vi "BMU诊断标定.vi"(5 "timeout":u32, 6 "Socket":dbl, 7 "通用配置?":bool, 8 "CAN端口":u16(ring), 9 "设备索引号":u16(ring), 10 "CAN卡类型":u32(ring)=21, 11 "从板号":u8=1) -> (3 "成功?":bool)   [LabVIEW 2013] (continued)
              n4251 = call "CAN_Init-8.6.vi"("CAN卡类型"=w6125, "设备索引号"=w6124, "CAN端口"=w6123, "操作类型"=enum16{"初始化CAN", "关闭CAN"}."初始化CAN", "滤波方式"=w6120, "Accept Code"=u32 3221225472, "簇"=T23 {"打开CAN"=FALSE, "初始化CAN"=TRUE, "开始CAN"=TRUE, "重启"=FALSE, "关闭CAN"=FALSE}, "Mask Code"=u32 1073741823 ("Accept Code"), "工作方式"=w6119, "是否滤波"=TRUE, "滤波选择"=T22 {"fiter_mode"=1, "fiter_endid"=402653184, "fiter_startid"=419430399}) -> ()  [unwired: 3 in, 6 out]
              n4252 = call <vilib>:"Unset Busy.vi"() -> ()  [unwired: 2 in, 10 out]
            }
          }
        }
        frame "强制均衡" {
          n4253 = local read "从板板号"() -> (w6129:u8)
          n4254 = stacked-sequence {
            tunnel: 133 -> [_ w6160 _ _]
            tunnel: w6129 -> [_ _ _ _]
            frame #0 {
              w6139 = u8 0 items=["Normal", "Listen Only"] ("工作方式")
              w6138 = u8 1 items=["Dual Filter", "Single Filter"] ("滤波方式")
              n4255 = global write "EV05全局变量1.vi" "读取超时"(FALSE ("读取超时")) -> ()
              n4256 = global write "EV05全局变量1.vi" "流控帧 2"(TRUE ("流控帧 2")) -> ()
              n4257 = local write "写?"(TRUE ("写?")) -> ()
              n4258 = local read "设备索引号"() -> (w6134:u16)
              n4259 = local read "CAN卡类型"() -> (w6133:u32)
              n4260 = local write "控制1"(TRUE ("控制1")) -> ()
              n4261 = local read "CAN端口"() -> (w6135:u16)
              n4262 = local write "消除"(TRUE ("消除")) -> ()
              n4263 = global write "EV05全局变量1.vi" "流控帧"(FALSE ("流控帧")) -> ()
              n4264 = call "CAN_Init-8.6.vi"("CAN卡类型"=w6133, "设备索引号"=w6134, "CAN端口"=w6135, "操作类型"=enum16{"初始化CAN", "关闭CAN"}."初始化CAN", "滤波方式"=w6138, "Accept Code"=u32 606601216, "簇"=T23 {"打开CAN"=FALSE, "初始化CAN"=TRUE, "开始CAN"=TRUE, "重启"=FALSE, "关闭CAN"=FALSE}, "Mask Code"=u32 524287 ("Accept Code"), "工作方式"=w6139, "是否滤波"=TRUE, "滤波选择"=T22 {"fiter_mode"=1, "fiter_endid"=75825152, "fiter_startid"=75890687}) -> ()  [unwired: 3 in, 6 out]
              n4265 = Wait Until Next ms Multiple(millisecond multiple=u32 20 ("毫秒倍数")) -> ()  [unwired: 1 out]
            }
            frame #1 {
              n4266 = local read "强制类型"() -> (w6166:enum16{"全通道开启", "单通道开启", "清待均衡时间"})
              n4267 = case shown="\"清待均衡时间\"" w6166 {
                tunnel: [250 252 254] -> w6156
                tunnel: [_ w6185 _] -> w6155
                tunnel: [_ w6184 _] -> w6154
                tunnel: [_ w6175 _] -> w6153
                tunnel: [_ w6168 _] -> w6152
                frame "全通道开启", Default {
                }
                frame "单通道开启" {
                  n4268 = local read "均衡类型选择"() -> (w6183:enum16{"放电均衡", "充电均衡", "充放电均衡"})
                  n4269 = local read "均衡位置"() -> (w6178:u16)
                  n4270 = case shown="\"放电均衡\", 默认" w6183 {
                    tunnel: [0 1] -> w6182
                    frame "放电均衡", Default {
                    }
                    frame "充电均衡" {
                    }
                  }
                  n4271 = Multiply(x="均衡时间", y=6.0) -> (x*y=w6170:dbl)
                  n4272 = Quotient & Remainder(x=w6170, y=256.0) -> (x-y*floor(x/y)=w6168:dbl, floor(x/y)=w6169:dbl)
                  n4273 = call "二进制解析-8.6.vi"("索引"=1, "数值"=w6182) -> ("低位子数组"=w6173:i32[])  [unwired: 1 in, 2 out]
                  n4274 = Quotient & Remainder(x=w6178, y=256.0) -> (x-y*floor(x/y)=w6184:dbl, floor(x/y)=w6185:dbl)
                  n4275 = call "二进制解析-8.6.vi"("索引"=8, "数值"=w6169) -> ("低位子数组"=w6174:i32[])  [unwired: 1 in, 2 out]
                  n4276 = Replace Array Subset(array=w6174, new element=w6173, index=0 ("索引")) -> (w6171:i32[])
                  n4277 = call "数值二进制转十进制-8.6.vi"("子数组"=w6171) -> ("十进制数值"=w6175:i32)  [unwired: 4 in]
                }
                frame "清待均衡时间" {
                }
              }
              n4278 = local write "命令"(w6160) -> ()
              n4279 = call "ID组合.vi"("SA(4)"=0 ("PDU(1)"), "PS(3)"=63 ("PDU(1)"), "PF(2)"=w6160, "PDU(1)"=4) -> ("ID"=w6159:i32)  [unwired: 7 out]
              n4280 = local read "设备索引号"() -> (w6163:u16)
              n4281 = local read "CAN卡类型"() -> (w6164:u32)
              n4282 = local read "CAN端口"() -> (w6162:u16)
              n4283 = local write "命令序号"(w6156) -> ()
              n4284 = Build Array(6, 4, w6156, w6155, w6154, w6153, w6152) -> (w6165:dbl[])
              n4285 = call "transmit-8.6.vi"("can卡类型"=w6164, "设备索引号"=w6163, "CAN端口"=w6162, "ID"=w6159, "SendType"=u8 0, "Data"=w6165) -> ()  [unwired: 3 in, 11 out]
            }
            frame #2 {
              n4286 = Wait Until Next ms Multiple(millisecond multiple=u32 1000 ("毫秒倍数")) -> ()  [unwired: 1 out]
            }
            frame #3 {
              w6199 = u8 0 items=["Normal", "Listen Only"] ("工作方式")
              w6198 = u8 1 items=["Dual Filter", "Single Filter"] ("滤波方式")
              n4287 = global write "EV05全局变量1.vi" "流控帧 2"(FALSE ("流控帧 2")) -> ()
              n4288 = local write "控制1"(FALSE ("控制1")) -> ()
              n4289 = local read "设备索引号"() -> (w6194:u16)
              n4290 = local read "CAN卡类型"() -> (w6193:u32)
              n4291 = local write "消除"(FALSE ("消除")) -> ()
              n4292 = local read "CAN端口"() -> (w6195:u16)
              n4293 = call <vilib>:"Unset Busy.vi"() -> ()  [unwired: 2 in, 10 out]
              n4294 = call "CAN_Init-8.6.vi"("CAN卡类型"=w6193, "设备索引号"=w6194, "CAN端口"=w6195, "操作类型"=enum16{"初始化CAN", "关闭CAN"}."初始化CAN", "滤波方式"=w6198, "Accept Code"=u32 3221225472, "簇"=T23 {"打开CAN"=FALSE, "初始化CAN"=TRUE, "开始CAN"=TRUE, "重启"=FALSE, "关闭CAN"=FALSE}, "Mask Code"=u32 1073741823 ("Accept Code"), "工作方式"=w6199, "是否滤波"=TRUE, "滤波选择"=T22 {"fiter_mode"=1, "fiter_endid"=402653184, "fiter_startid"=419430399}) -> ()  [unwired: 3 in, 6 out]
            }
          }
        }
        frame "项目软件版本读取" {
          n4295 = stacked-sequence {
            seq-local: [_ w6220 _] -> [_ _ w6227]
            frame #0 {
              n4296 = local read "设备索引号"() -> (w6207:u16)
              n4297 = local read "CAN卡类型"() -> (w6208:u32)
              n4298 = local read "CAN端口"() -> (w6206:u16)
              n4299 = stacked-sequence {
                tunnel: w6208 -> [w6211 w6219]
                tunnel: w6207 -> [w6210 w6218]
                tunnel: w6206 -> [w6209 w6217]
                frame #0 {
                  n4300 = dll-call lib="PTH1abs FBluewave New EnergySVN_WorkAutoTest_TestStandtrunkAutoTest_TestStandDriverZlgCanBHN01è¯»ååæ°data\nkerneldlls\nusbcan.dll" fn="VCI_ClearBuffer"("DeviceType"=w6211, "DeviceInd"=w6210, "CANInd"=w6209) -> (error out=w6212:errorcluster)  [unwired: 4 in, 4 out]
                  n4301 = call <vilib>:"Clear Errors.vi"("error in (no error)"=w6212) -> ()  [unwired: 6 in, 1 out]
                }
                frame #1 {
                  w6216 = u8 137 ("命令")
                  w6215 = u32 1 ("命令序号")
                  n4302 = local read "从板板号"() -> (w6213:u8)
                  n4303 = local write "命令"(w6216) -> ()
                  n4304 = call "多帧发送机制(EV05).vi"("can卡类型"=w6219, "设备索引号"=w6218, "CAN端口"=w6217, "命令"=w6216, "板号"=w6213, "命令序号"=w6215, "输入数据"=dbl[] [0.0]) -> ()  [unwired: 2 in, 11 out]
                  n4305 = local write "命令序号"(w6215) -> ()
                }
              }
            }
            frame #1 {
              n4306 = while {
                tunnel: [w6221] -> w6220
                i -> [w6226]
                stop <- w6223 stop-if-true
                n4307 = global read "EV05全局变量1.vi" "写入超时"() -> (w6221:bool)
                n4308 = Greater Or Equal?(x=w6226, y=25) -> (x >= y?=w6224:bool)
                n4309 = Or(x=w6221, y=w6224) -> (x .or. y?=w6223:bool)
                n4310 = Wait Until Next ms Multiple(millisecond multiple=u32 100 ("毫秒倍数")) -> ()  [unwired: 1 out]
              }
            }
            frame #2 {
              n4311 = case shown="假" w6227 {
                frame False {
                  n4312 = control-ref of="结果"() -> (w6229:refnum<vi>)
                  n4313 = Concatenate Strings("项目软件版本" ("字符串"), "     读取失败" ("字符串")) -> (w6232:string)
                  n4314 = Build Array(w6232) -> (w6231:string[])
                  n4315 = call "表格编辑(版本读取).vi"("新元素/子数组"=w6231, "活动单元格:单元格背景色"=u32 16740749, "MCListbox引用句柄"=w6229) -> ()  [unwired: 9 out]
                }
                frame True {
                }
              }
              n4316 = call <vilib>:"Unset Busy.vi"() -> ()  [unwired: 2 in, 10 out]
            }
          }
        }
        frame "读取故障状态" {
          n4317 = stacked-sequence {
            seq-local: [_ w6258 _] -> [_ _ w6265]
            frame #0 {
              n4318 = local read "设备索引号"() -> (w6235:u16)
              n4319 = local read "CAN卡类型"() -> (w6236:u32)
              n4320 = local read "CAN端口"() -> (w6234:u16)
              n4321 = stacked-sequence {
                tunnel: w6236 -> [w6239 w6248]
                tunnel: w6235 -> [w6238 w6247]
                tunnel: w6234 -> [w6237 w6246]
                frame #0 {
                  n4322 = dll-call lib="PTH1abs FBluewave New EnergySVN_WorkAutoTest_TestStandtrunkAutoTest_TestStandDriverZlgCanBHN01è¯»ååæ°data\nkerneldlls\nusbcan.dll" fn="VCI_ClearBuffer"("DeviceType"=w6239, "DeviceInd"=w6238, "CANInd"=w6237) -> (error out=w6240:errorcluster)  [unwired: 4 in, 4 out]
                  n4323 = call <vilib>:"Clear Errors.vi"("error in (no error)"=w6240) -> ()  [unwired: 6 in, 1 out]
                }
                frame #1 {
                  n4324 = local read "从板板号 2"() -> (w6241:u8)
                  n4325 = case shown="1..30" w6241 {
                    tunnel: [u8 133 ("命令") u8 4 ("命令")] -> w6245
                    frame 0, Default {
                    }
                    frame 1..30 {
                    }
                  }
                  n4326 = local read "状态选择"() -> (w6243:T18)
                  n4327 = local write "命令"(w6245) -> ()
                  n4328 = case shown="\"预充电故障,继电器驱动故障\"" w6243 {
                    tunnel: [1 2 3 4 5 6 7] -> w6242
                    frame "电压,内总电压,外总电压,温度,电流,绝缘,系统时钟,充电均衡,放电均衡", Default {
                    }
                    frame "CPU,CPU内部EE存储器,CPU内部FLASH,内部EE存储器,45db存储器" {
                    }
                    frame "CAN检测故障" {
                    }
                    frame "软件故障" {
                    }
                    frame "RS485,RS232检测故障" {
                    }
                    frame "DI,DO,AI,AO检测故障" {
                    }
                    frame "预充电故障,继电器驱动故障" {
                    }
                  }
                  n4329 = call "多帧发送机制(EV05).vi"("can卡类型"=w6248, "设备索引号"=w6247, "CAN端口"=w6246, "命令"=w6245, "板号"=w6241, "命令序号"=w6242, "输入数据"=dbl[] [0.0]) -> ()  [unwired: 2 in, 11 out]
                  n4330 = local write "命令序号"(w6242) -> ()
                }
              }
            }
            frame #1 {
              n4331 = while {
                tunnel: [w6259] -> w6258
                i -> [w6264]
                stop <- w6261 stop-if-true
                n4332 = global read "EV05全局变量1.vi" "写入超时"() -> (w6259:bool)
                n4333 = Greater Or Equal?(x=w6264, y=25) -> (x >= y?=w6262:bool)
                n4334 = Or(x=w6259, y=w6262) -> (x .or. y?=w6261:bool)
                n4335 = Wait Until Next ms Multiple(millisecond multiple=u32 100 ("毫秒倍数")) -> ()  [unwired: 1 out]
              }
            }
            frame #2 {
              n4336 = case shown="真" w6265 {
                frame False {
                  n4337 = Concatenate Strings("故障信息" ("字符串"), "     读取失败" ("字符串")) -> (w6267:string)
                  n4338 = One Button Dialog(message=w6267, button name ("OK")="确定" ("按钮名称（“确定”）")) -> ()  [unwired: 1 out]
                }
                frame True {
                  n4339 = One Button Dialog(message="故障信息读取完成" ("字符串"), button name ("OK")="确定" ("按钮名称（“确定”）")) -> ()  [unwired: 1 out]
                }
              }
              n4340 = call <vilib>:"Unset Busy.vi"() -> ()  [unwired: 2 in, 10 out]
            }
          }
        }
        frame "平台软件版本读取" {
          n4341 = stacked-sequence {
            seq-local: [_ w6287 _] -> [_ _ w6294]
            frame #0 {
              n4342 = local read "设备索引号"() -> (w6274:u16)
              n4343 = local read "CAN卡类型"() -> (w6275:u32)
              n4344 = local read "CAN端口"() -> (w6273:u16)
              n4345 = stacked-sequence {
                tunnel: w6275 -> [w6278 w6286]
                tunnel: w6274 -> [w6277 w6285]
                tunnel: w6273 -> [w6276 w6284]
                tunnel: u8 137 ("命令") -> [_ w6283]
                frame #0 {
                  n4346 = dll-call lib="PTH1abs FBluewave New EnergySVN_WorkAutoTest_TestStandtrunkAutoTest_TestStandDriverZlgCanBHN01è¯»ååæ°data\nkerneldlls\nusbcan.dll" fn="VCI_ClearBuffer"("DeviceType"=w6278, "DeviceInd"=w6277, "CANInd"=w6276) -> (error out=w6279:errorcluster)  [unwired: 4 in, 4 out]
                  n4347 = call <vilib>:"Clear Errors.vi"("error in (no error)"=w6279) -> ()  [unwired: 6 in, 1 out]
                }
                frame #1 {
                  w6282 = u32 2 ("命令序号")
                  n4348 = local read "从板板号"() -> (w6280:u8)
                  n4349 = local write "命令"(w6283) -> ()
                  n4350 = call "多帧发送机制(EV05).vi"("can卡类型"=w6286, "设备索引号"=w6285, "CAN端口"=w6284, "命令"=w6283, "板号"=w6280, "命令序号"=w6282, "输入数据"=dbl[] [0.0]) -> ()  [unwired: 2 in, 11 out]
                  n4351 = local write "命令序号"(w6282) -> ()
                }
              }
            }
            frame #1 {
              n4352 = while {
                tunnel: [w6288] -> w6287
                i -> [w6293]
                stop <- w6290 stop-if-true
                n4353 = global read "EV05全局变量1.vi" "写入超时"() -> (w6288:bool)
                n4354 = Greater Or Equal?(x=w6293, y=25) -> (x >= y?=w6291:bool)
                n4355 = Or(x=w6288, y=w6291) -> (x .or. y?=w6290:bool)
                n4356 = Wait Until Next ms Multiple(millisecond multiple=u32 100 ("毫秒倍数")) -> ()  [unwired: 1 out]
              }
            }
            frame #2 {
              n4357 = case shown="假" w6294 {
                frame False {
                  n4358 = control-ref of="结果"() -> (w6297:refnum<vi>)
                  n4359 = Concatenate Strings("平台软件版本" ("字符串"), "     读取失败" ("字符串")) -> (w6299:string)
                  n4360 = Build Array(w6299) -> (w6296:string[])
                  n4361 = call "表格编辑(版本读取).vi"("新元素/子数组"=w6296, "活动单元格:单元格背景色"=u32 16740749, "MCListbox引用句柄"=w6297) -> ()  [unwired: 9 out]
                }
                frame True {
                }
              }
              n4362 = call <vilib>:"Unset Busy.vi"() -> ()  [unwired: 2 in, 10 out]
            }
          }
        }
        frame "模块软件版本读取" {
          n4363 = local read "从板板号"() -> (w6301:u8)
          n4364 = local read "模块软件版本"() -> (w6302:T1)
          n4365 = case shown="\"全部读取\"" w6302 {
            selector: w6302 -> [w6303 w6347]
            tunnel: w6301 -> [_ w6346]
            frame "BCUMCAL", Default {
              n4366 = stacked-sequence {
                seq-local: [_ _ w6329 _] -> [_ _ _ w6336]
                tunnel: w6303 -> [_ w6309 _ w6337]
                frame #0 {
                  w6308 = FALSE ("写?")
                  n4367 = call <vilib>:"Set Busy.vi"("disable click? (T)"=FALSE) -> ()  [unwired: 3 in, 8 out]
                  n4368 = local write "写?"(w6308) -> ()
                  n4369 = global write "EV05全局变量1.vi" "流控帧 2"(TRUE ("流控帧 2")) -> ()
                  n4370 = global write "EV05全局变量1.vi" "写入超时"(w6308) -> ()
                  n4371 = local write "控制1"(TRUE ("控制1")) -> ()
                  n4372 = local write "消除"(TRUE ("消除")) -> ()
                }
                frame #1 {
                  n4373 = Quotient & Remainder(x=w6309, y=256) -> (x-y*floor(x/y)=w6310:i32, floor(x/y)=w6311:i32)
                  n4374 = Build Array(w6311, w6310, u8 0 ("板号")) -> (w6314:i32[])
                  n4375 = local read "设备索引号"() -> (w6316:u16)
                  n4376 = local read "CAN卡类型"() -> (w6317:u32)
                  n4377 = local read "CAN端口"() -> (w6315:u16)
                  n4378 = stacked-sequence {
                    tunnel: w6317 -> [w6320 w6328]
                    tunnel: w6316 -> [w6319 w6327]
                    tunnel: w6315 -> [w6318 w6326]
                    tunnel: w6314 -> [_ w6325]
                    frame #0 {
                      n4379 = dll-call lib="PTH1abs FBluewave New EnergySVN_WorkAutoTest_TestStandtrunkAutoTest_TestStandDriverZlgCanBHN01è¯»ååæ°data\nkerneldlls\nusbcan.dll" fn="VCI_ClearBuffer"("DeviceType"=w6320, "DeviceInd"=w6319, "CANInd"=w6318) -> (error out=w6321:errorcluster)  [unwired: 4 in, 4 out]
                      n4380 = call <vilib>:"Clear Errors.vi"("error in (no error)"=w6321) -> ()  [unwired: 6 in, 1 out]
                    }
                    frame #1 {
                      w6324 = u8 137 ("命令")
                      w6322 = u32 3 ("命令序号")
                      n4381 = local read "从板板号"() -> (w6323:u8)
                      n4382 = local write "命令"(w6324) -> ()
                      n4383 = call "多帧发送机制(EV05).vi"("can卡类型"=w6328, "设备索引号"=w6327, "CAN端口"=w6326, "命令"=w6324, "板号"=w6323, "命令序号"=w6322, "输入数据"=w6325) -> ()  [unwired: 2 in, 11 out]
                      n4384 = local write "命令序号"(w6322) -> ()
                    }
                  }
                }
                frame #2 {
                  n4385 = while {
                    tunnel: [w6330] -> w6329
                    i -> [w6335]
                    stop <- w6331 stop-if-true
                    n4386 = global read "EV05全局变量1.vi" "写入超时"() -> (w6330:bool)
                    n4387 = Greater Or Equal?(x=w6335, y=25) -> (x >= y?=w6332:bool)
                    n4388 = Or(x=w6330, y=w6332) -> (x .or. y?=w6331:bool)
                    n4389 = Wait Until Next ms Multiple(millisecond multiple=u32 100 ("毫秒倍数")) -> ()  [unwired: 1 out]
                  }
                }
                frame #3 {
                  n4390 = call <vilib>:"Unset Busy.vi"() -> ()  [unwired: 2 in, 10 out]
                  n4391 = case shown="假" w6336 {
                    tunnel: w6337 -> [w6339 _]
                    frame False {
                      n4392 = Number To Decimal String(number=w6339) -> (decimal integer string=w6340:string)  [unwired: 1 out]
                      n4393 = control-ref of="结果"() -> (w6341:refnum<vi>)
                      n4394 = Concatenate Strings("模块" ("字符串"), w6340, "     读取失败" ("字符串")) -> (w6344:string)
                      n4395 = Build Array(w6344) -> (w6343:string[])
                      n4396 = call "表格编辑(版本读取).vi"("新元素/子数组"=w6343, "活动单元格:单元格背景色"=u32 16740749, "MCListbox引用句柄"=w6341) -> ()  [unwired: 9 out]
                    }
                    frame True {
                    }
                  }
                }
              }
            }
            frame "全部读取" {
              n4397 = stacked-sequence {
                seq-local: [w6348 _] -> [_ w6386]
                tunnel: w6347 -> [_ w6388]
                tunnel: w6346 -> [w6349 w6387]
                frame #0 {
                  n4398 = stacked-sequence {
                    tunnel: w6349 -> [_ w6358 _]
                    tunnel: [_ _ w6378] -> w6348
                    frame #0 {
                      w6354 = FALSE ("写?")
                      n4399 = control-ref of="模块软件版本 2"() -> (w6352:refnum<vi>)
                      n4400 = call <vilib>:"Set Busy.vi"("disable click? (T)"=FALSE) -> ()  [unwired: 3 in, 8 out]
                      n4401 = local write "写?"(w6354) -> ()
                      n4402 = property class="MCListbox (严格)"(reference=w6352, "ItemNames"=string[][] []) -> ()  [unwired: 1 in, 2 out]
                      n4403 = global write "EV05全局变量1.vi" "写入超时"(w6354) -> ()
                      n4404 = local write "消除"(TRUE ("消除")) -> ()
                      n4405 = global write "EV05全局变量1.vi" "流控帧 2"(TRUE ("流控帧 2")) -> ()
                      n4406 = local write "控制1"(TRUE ("控制1")) -> ()
                      n4407 = local write "MODEL号"(u8[] [] ("MODEL号")) -> ()
                    }
                    frame #1 {
                      n4408 = local read "设备索引号"() -> (w6360:u16)
                      n4409 = local read "CAN卡类型"() -> (w6361:u32)
                      n4410 = local read "CAN端口"() -> (w6359:u16)
                      n4411 = stacked-sequence {
                        tunnel: w6361 -> [w6364 w6377]
                        tunnel: w6360 -> [w6363 w6376]
                        tunnel: w6359 -> [w6362 w6375]
                        tunnel: w6358 -> [_ w6367]
                        frame #0 {
                          n4412 = dll-call lib="PTH1abs FBluewave New EnergySVN_WorkAutoTest_TestStandtrunkAutoTest_TestStandDriverZlgCanBHN01è¯»ååæ°data\nkerneldlls\nusbcan.dll" fn="VCI_ClearBuffer"("DeviceType"=w6364, "DeviceInd"=w6363, "CANInd"=w6362) -> (error out=w6365:errorcluster)  [unwired: 4 in, 4 out]
                          n4413 = call <vilib>:"Clear Errors.vi"("error in (no error)"=w6365) -> ()  [unwired: 6 in, 1 out]
                        }
                        frame #1 {
                          w6373 = u8 137 ("命令")
                          w6371 = u32 3 ("命令序号")
                          n4414 = Quotient & Remainder(x=u8 0 ("板号"), y=256) -> (x-y*floor(x/y)=w6368:i32, floor(x/y)=w6369:i32)
                          n4415 = local write "命令"(w6373) -> ()
                          n4416 = Build Array(w6369, w6368, u8 0 ("板号")) -> (w6374:i32[])
                          n4417 = call "多帧发送机制(EV05).vi"("can卡类型"=w6377, "设备索引号"=w6376, "CAN端口"=w6375, "命令"=w6373, "板号"=w6367, "命令序号"=w6371, "输入数据"=w6374) -> ()  [unwired: 2 in, 11 out]
                          n4418 = local write "命令序号"(w6371) -> ()
                        }
                      }
                    }
                    frame #2 {
                      n4419 = while {
                        tunnel: [w6380] -> w6378
                        i -> [w6384]
                        stop <- w6381 stop-if-true
                        n4420 = local read "强制停止版本读取"() -> (w6379:bool)
                        n4421 = global read "EV05全局变量1.vi" "写入超时"() -> (w6380:bool)
                        n4422 = Greater Or Equal?(x=w6384, y=35) -> (x >= y?=w6382:bool)
                        n4423 = Compound Arithmetic op=OR(w6379, w6380, w6382) -> (w6381:bool)
                        n4424 = Wait Until Next ms Multiple(millisecond multiple=u32 100 ("毫秒倍数")) -> ()  [unwired: 1 out]
                      }
                    }
                  }
                }
                frame #1 {
                  n4425 = case shown="真" w6386 {
                    tunnel: w6388 -> [_ w6398]
                    tunnel: w6387 -> [_ w6397]
                    frame False {
                      n4426 = control-ref of="结果"() -> (w6390:refnum<vi>)
                      n4427 = Concatenate Strings("模块编号" ("字符串"), "读取失败" ("字符串")) -> (w6393:string)
                      n4428 = Build Array(w6393) -> (w6392:string[])
                      n4429 = call "表格编辑(版本读取).vi"("新元素/子数组"=w6392, "活动单元格:单元格背景色"=u32 16740749, "MCListbox引用句柄"=w6390) -> ()  [unwired: 9 out]
                      n4430 = call <vilib>:"Unset Busy.vi"() -> ()  [unwired: 11 in, 1 out]
                    }
                    frame True {
                      n4431 = local read "MODEL号"() -> (w6396:u8[])
                      n4432 = Array Size(array=w6396) -> (size(s)=w6395:i32)
                      n4433 = for {
                        tunnel: w6398 -> [_]
                        tunnel: w6397 -> [w6401]
                        tunnel: w6396 -> [w6400] mode=indexing
                        tunnel: w6395 -> [w6399]
                        i -> [w6403]
                        n4434 = Increment(x=w6403) -> (x+1=w6402:i32)
                        n4435 = stacked-sequence {
                          seq-local: [_ _ _ w6430 _ _] -> [_ _ _ _ w6439 _]
                          seq-local: [_ w6409 _ _ _ _] -> [_ _ _ _ w6438 _]
                          tunnel: w6402 -> [_ _ _ _ _ w6450]
                          tunnel: w6400 -> [_ w6409 _ _ _ _]
                          tunnel: w6401 -> [_ w6410 _ _ _ _]
                          tunnel: w6399 -> [_ _ _ _ _ w6448]
                          frame #0 {
                            w6405 = FALSE ("写?")
                            n4436 = call <vilib>:"Set Busy.vi"("disable click? (T)"=FALSE) -> ()  [unwired: 3 in, 8 out]
                            n4437 = local write "写?"(w6405) -> ()
                            n4438 = global write "EV05全局变量1.vi" "写入超时"(w6405) -> ()
                            n4439 = global write "EV05全局变量1.vi" "流控帧 2"(TRUE ("流控帧 2")) -> ()
                            n4440 = local write "控制1"(TRUE ("控制1")) -> ()
                            n4441 = local write "消除"(TRUE ("消除")) -> ()
                          }
                          frame #1 {
                            n4442 = local read "设备索引号"() -> (w6412:u16)
                            n4443 = local read "CAN卡类型"() -> (w6413:u32)
                            n4444 = local read "CAN端口"() -> (w6411:u16)
                            n4445 = stacked-sequence {
                              tunnel: w6413 -> [w6416 w6429]
                              tunnel: w6412 -> [w6415 w6428]
                              tunnel: w6411 -> [w6414 w6427]
                              tunnel: w6410 -> [_ w6419]
                              tunnel: w6409 -> [_ w6418]
                              frame #0 {
                                n4446 = dll-call lib="PTH1abs FBluewave New EnergySVN_WorkAutoTest_TestStandtrunkAutoTest_TestStandDriverZlgCanBHN01è¯»ååæ°data\nkerneldlls\nusbcan.dll" fn="VCI_ClearBuffer"("DeviceType"=w6416, "DeviceInd"=w6415, "CANInd"=w6414) -> (error out=w6417:errorcluster)  [unwired: 4 in, 4 out]
                                n4447 = call <vilib>:"Clear Errors.vi"("error in (no error)"=w6417) -> ()  [unwired: 6 in, 1 out]
                              }
                              frame #1 {
                                w6425 = u8 137 ("命令")
                                w6423 = u32 3 ("命令序号")
                                n4448 = Quotient & Remainder(x=w6418, y=256) -> (x-y*floor(x/y)=w6420:i32, floor(x/y)=w6421:i32)
                                n4449 = local write "命令"(w6425) -> ()
                                n4450 = Build Array(w6421, w6420, u8 0 ("板号")) -> (w6426:i32[])
                                n4451 = call "多帧发送机制(EV05).vi"("can卡类型"=w6429, "设备索引号"=w6428, "CAN端口"=w6427, "命令"=w6425, "板号"=w6419, "命令序号"=w6423, "输入数据"=w6426) -> ()  [unwired: 2 in, 11 out]
                                n4452 = local write "命令序号"(w6423) -> ()
                              }
                            }
                          }
                          frame #2 {
                          }
                          frame #3 {
                            n4453 = while {
                              tunnel: [w6432] -> w6430
                              i -> [w6436]
                              stop <- w6433 stop-if-true
                              n4454 = local read "强制停止版本读取"() -> (w6431:bool)
                              n4455 = global read "EV05全局变量1.vi" "写入超时"() -> (w6432:bool)
                              n4456 = Greater Or Equal?(x=w6436, y=25) -> (x >= y?=w6434:bool)
                              n4457 = Compound Arithmetic op=OR(w6431, w6432, w6434) -> (w6433:bool)
                              n4458 = Wait Until Next ms Multiple(millisecond multiple=u32 100 ("毫秒倍数")) -> ()  [unwired: 1 out]
                            }
                          }
                          frame #4 {
                            n4459 = call <vilib>:"Unset Busy.vi"() -> ()  [unwired: 11 in, 1 out]
                            n4460 = case shown="假" w6439 {
                              tunnel: w6438 -> [w6441 _]
                              frame False {
                                n4461 = control-ref of="结果"() -> (w6443:refnum<vi>)
                                n4462 = Number To Decimal String(number=w6441) -> (decimal integer string=w6442:string)  [unwired: 1 out]
                                n4463 = Concatenate Strings("模块" ("字符串"), w6442, "     读取失败" ("字符串")) -> (w6446:string)
                                n4464 = Build Array(w6446) -> (w6445:string[])
                                n4465 = call "表格编辑(版本读取).vi"("新元素/子数组"=w6445, "活动单元格:单元格背景色"=u32 16740749, "MCListbox引用句柄"=w6443) -> ()  [unwired: 9 out]
                              }
                              frame True {
                              }
                            }
                          }
                          frame #5 {
                            n4466 = Equal?(x=w6448, y=w6450) -> (x = y?=w6449:bool)
                            n4467 = case shown="真" w6449 {
                              frame False {
                              }
                              frame True {
                                n4468 = control-ref of="模块软件版本 2"() -> (w6461:refnum<vi>)
                                n4469 = local read "模块版本名称"() -> (w6460:string[][])
                                n4470 = local read "模块版本值"() -> (w6456:string[][])
                                n4471 = control-ref of="结果"() -> (w6468:refnum<vi>)
                                n4472 = property class="MCListbox (严格)"(reference=w6461) -> ("ItemNames"=w6464:string[][])  [unwired: 1 in, 2 out]
                                n4473 = local read "从板板号"() -> (w6451:u8)
                                n4474 = Concatenate Strings("模块版本读取完成" ("字符串")) -> (w6471:string)
                                n4475 = Build Array(w6471) -> (w6470:string[])
                                n4476 = call "表格编辑(版本读取).vi"("新元素/子数组"=w6470, "活动单元格:单元格背景色"=u32 21937, "MCListbox引用句柄"=w6468) -> ()  [unwired: 9 out]
                                n4477 = Transpose 2D Array(2D array=w6464) -> (transposed array=w6465:string[][])
                                n4478 = local write "强制停止版本读取"(FALSE ("强制停止 2")) -> ()
                                n4479 = local read "模块个数"() -> (w6454:u8[])
                                n4480 = Index Array(array=w6465, index (row) #1=0 ("索引 (行)"), index (row) #2=1 ("索引 (行)")) -> (element #1=w6455:string[], element #2=w6457:string[])  [unwired: 2 in]
                                n4481 = Replace Array Subset(array=w6460, new element=w6455, index (row)=w6451) -> (w6459:string[][])  [unwired: 1 in]
                                n4482 = Replace Array Subset(array=w6456, new element=w6457, index (row)=w6451) -> (w6458:string[][])  [unwired: 1 in]
                                n4483 = local write "模块版本名称"(w6459) -> ()
                                n4484 = local write "模块版本值"(w6458) -> ()
                                n4485 = Array Size(array=w6455) -> (size(s)=w6452:i32)
                                n4486 = Replace Array Subset(array=w6454, new element=w6452, index=w6451) -> (w6453:u8[])
                                n4487 = local write "模块个数"(w6453) -> ()
                              }
                            }
                          }
                        }
                      }
                    }
                  }
                }
              }
            }
          }
        }
        frame "硬件版本读取" {
          n4488 = stacked-sequence {
            seq-local: [_ _ w6479 _] -> [_ _ _ w6486]
            frame #0 {
              w6475 = u8 137 ("命令")
              w6474 = u32 4 ("命令序号")
              n4489 = local read "设备索引号"() -> (w6477:u16)
              n4490 = local read "CAN卡类型"() -> (w6478:u32)
              n4491 = local read "CAN端口"() -> (w6476:u16)
              n4492 = local read "从板板号"() -> (w6472:u8)
              n4493 = local write "命令"(w6475) -> ()
              n4494 = call "多帧发送机制(EV05).vi"("can卡类型"=w6478, "设备索引号"=w6477, "CAN端口"=w6476, "命令"=w6475, "板号"=w6472, "命令序号"=w6474, "输入数据"=dbl[] [0.0]) -> ()  [unwired: 2 in, 11 out]
              n4495 = local write "命令序号"(w6474) -> ()
            }
            frame #1 {
            }
            frame #2 {
              n4496 = while {
                tunnel: [w6480] -> w6479
                i -> [w6485]
                stop <- w6481 stop-if-true
                n4497 = global read "EV05全局变量1.vi" "写入超时"() -> (w6480:bool)
                n4498 = Greater Or Equal?(x=w6485, y=25) -> (x >= y?=w6482:bool)
                n4499 = Or(x=w6480, y=w6482) -> (x .or. y?=w6481:bool)
                n4500 = Wait Until Next ms Multiple(millisecond multiple=u32 100 ("毫秒倍数")) -> ()  [unwired: 1 out]
              }
            }
            frame #3 {
              n4501 = case shown="假" w6486 {
                frame False {
                  n4502 = control-ref of="结果"() -> (w6488:refnum<vi>)
                  n4503 = Concatenate Strings("硬件版本" ("字符串"), "     读取失败" ("字符串")) -> (w6491:string)
                  n4504 = Build Array(w6491) -> (w6490:string[])
                  n4505 = call "表格编辑(版本读取).vi"("新元素/子数组"=w6490, "活动单元格:单元格背景色"=u32 16740749, "MCListbox引用句柄"=w6488) -> ()  [unwired: 9 out]
                }
                frame True {
                }
              }
              n4506 = call <vilib>:"Unset Busy.vi"() -> ()  [unwired: 2 in, 10 out]
            }
          }
        }
        frame "写配置文件" {
          n4507 = disable-structure shown="启用" {
            frame Enabled {
              n4508 = local read "主从选择"() -> (w6499:enum32{"主板", "从板"})
              n4509 = case shown="\"从板\"" w6499 {
                tunnel: [w6518 w6709] -> w6502
                tunnel: ["M0" w6715] -> w6500
                frame "主板", Default {
                  n4510 = stacked-sequence {
                    seq-local: [w6532 _ _ _ _ _ _] -> [_ w6561 _ _ _ _ _]
                    seq-local: [string[] ["电池额定容量", "电池实际容量", "SOC", "SOH", "车牌号", "配置文件版本", "产品编号", "系统时钟"] _ _ _ _ _ _] -> [_ w6556 _ _ _ _ _]
                    seq-local: [_ _ _ _ string[] ["风机开启温度", "风机关闭温度", "加热开启温度", "加热关闭温度", "风机开启温差", "风机关闭温差", "加热关闭温差"] _ _] -> [_ _ _ _ _ w6661 _]
                    seq-local: [_ _ _ _ w6642 _ _] -> [_ _ _ _ _ w6659 _]
                    tunnel: [w6533 _ _ _ _ _ _] -> w6520
                    tunnel: [_ w6563 _ _ _ _ _] -> w6517
                    tunnel: [_ _ w6587 _ _ _ _] -> w6516
                    tunnel: [_ _ _ w6614 _ _ _] -> w6515
                    tunnel: [_ _ _ _ _ w6662 _] -> w6514
                    tunnel: [_ _ _ _ _ _ w6679] -> w6513
                    frame #0 {
                      w6524 = string[] ["", "", "", "", "", "", "", "", "", "", "  "]
                      n4511 = control-ref of="项目信息"() -> (w6552:refnum<vi>)
                      n4512 = property class="Tbl (严格)"(reference=w6552) -> ("Value"=w6528:string[][])  [unwired: 1 in, 2 out]
                      n4513 = control-ref of="项目信息2"() -> (w6546:refnum<vi>)
                      n4514 = Index Array(array=w6528, index (col)=0 ("禁用的索引 (列)")) -> (element=w6529:string[])  [unwired: 1 in]
                      n4515 = property class="Clust (严格)"(reference=w6546) -> ("Value"=w6545:T9)  [unwired: 1 in, 2 out]
                      n4516 = Index Array(array=w6528, index (col)=1 ("禁用的索引 (列)")) -> (element=w6527:string[])  [unwired: 1 in]
                      n4517 = local read "从板个数"() -> (w6551:dbl)
                      n4518 = Number To Decimal String(number=w6551) -> (decimal integer string=w6550:string)  [unwired: 1 out]
                      n4519 = Insert Into Array(array=w6529, new element=w6524) -> (w6526:string[])  [unwired: 1 in]
                      n4520 = Insert Into Array(array=w6527, new element=w6524) -> (w6525:string[])  [unwired: 1 in]
                      n4521 = Unbundle(w6545) -> ("电池额定容量(A)"=w6544:dbl, "电池实际容量(A)"=w6543:dbl, "车架(牌)号"=w6541:string, "配置文件版本"=w6540:string, "SOH(%)"=w6535:dbl, "SOC(%)"=w6534:dbl, "产品编号"=w6539:string, "系统时钟"=w6538:string)  [unwired: 1 out]
                      n4522 = Build Array("从板个数" ("元素"), w6550) -> (w6547:string[])
                      n4523 = Build Array(w6526, w6525) -> (w6522:string[][])
                      n4524 = Transpose 2D Array(2D array=w6522) -> (transposed array=w6521:string[][])
                      n4525 = Build Array(w6544, w6543, w6534, w6535) -> (w6542:dbl[])
                      n4526 = Build Array(w6541, w6540, w6539, w6538) -> (w6536:string[])
                      n4527 = for {
                        tunnel: w6542 -> [w6554] mode=indexing
                        tunnel: [w6553] -> w6537 mode=indexing
                        n4528 = Format Into String(format string="%#f" ("格式字符串"), w6554) -> (resulting string=w6553:string)  [unwired: 2 in, 1 out]
                      }
                      n4529 = Insert Into Array(array=w6521, index (row)=0 ("索引 (行)"), new element=w6547) -> (w6533:string[][])  [unwired: 1 in]
                      n4530 = Insert Into Array(array=w6537, new element=w6536) -> (w6532:string[])  [unwired: 1 in]
                    }
                    frame #1 {
                      n4531 = control-ref of="一级故障"() -> (w6583:refnum<vi>)
                      n4532 = property class="Clust (严格)"(reference=w6583) -> ("Value"=w6582:T10)  [unwired: 1 in, 2 out]
                      n4533 = Unbundle(w6582) -> ("总电压过高"=w6581:dbl, "整组电压不均衡"=w6576:dbl, "SOC过高"=w6569:dbl, "单体电压过高"=w6572:dbl, "总电压过低"=w6580:dbl, "温度过高"=w6579:dbl, "温度过低"=w6578:dbl, "单组电压不均衡"=w6577:dbl, "整组温度不均衡"=w6574:dbl, "单组温度不均衡"=w6575:dbl, "单体电压过低"=w6573:dbl, "充电电流过高"=w6571:dbl, "放电电流过高"=w6570:dbl, "SOC过低"=w6568:dbl, "内阻过大"=w6567:dbl, "极柱温度过高"=w6566:dbl, "SOH过低"=w6565:dbl)
                      n4534 = Build Array(w6581, w6580, w6579, w6578, w6577, w6576, w6575, w6574, w6572, w6573, w6571, w6570, w6569, w6568, w6567, w6566, w6565) -> (w6564:dbl[])
                      n4535 = for {
                        tunnel: w6564 -> [w6585] mode=indexing
                        tunnel: [w6584] -> w6560 mode=indexing
                        n4536 = Format Into String(format string="%#f" ("格式字符串"), w6585) -> (resulting string=w6584:string)  [unwired: 2 in, 1 out]
                      }
                      n4537 = Insert Into Array(array=w6561, new element=w6560) -> (w6559:string[])  [unwired: 1 in]
                      n4538 = Insert Into Array(array=w6556, new element=string[] ["总电压过高一级", "总电压过低一级", "温度过高一级", "温度过低一级", "单组电压不均衡一级", "整组电压不均衡一级", "单组温度不均衡一级", "整组温度不均衡一级", "单体电压过高一级", "单体电压过低一级", "充电电流过高一级", "放电电流过高一级", "SOC过高一级", "SOC过低一级", "内阻过大一级", "极柱温度过高一级", "SOH过低一级"]) -> (w6558:string[])  [unwired: 1 in]
                      n4539 = Build Array(w6558, w6559) -> (w6557:string[][])
                      n4540 = Transpose 2D Array(2D array=w6557) -> (transposed array=w6563:string[][])
                    }
                    frame #2 {
                      n4541 = control-ref of="一级故障 2"() -> (w6588:refnum<vi>)
                      n4542 = property class="Clust (严格)"(reference=w6588) -> ("Value"=w6610:T10)  [unwired: 1 in, 2 out]
                      n4543 = Unbundle(w6610) -> ("总电压过高"=w6609:dbl, "整组电压不均衡"=w6604:dbl, "SOC过高"=w6597:dbl, "单体电压过高"=w6600:dbl, "总电压过低"=w6608:dbl, "温度过高"=w6607:dbl, "温度过低"=w6606:dbl, "单组电压不均衡"=w6605:dbl, "整组温度不均衡"=w6602:dbl, "单组温度不均衡"=w6603:dbl, "单体电压过低"=w6601:dbl, "充电电流过高"=w6599:dbl, "放电电流过高"=w6598:dbl, "SOC过低"=w6596:dbl, "内阻过大"=w6595:dbl, "极柱温度过高"=w6594:dbl, "SOH过低"=w6593:dbl)
                      n4544 = Build Array(w6609, w6608, w6607, w6606, w6605, w6604, w6603, w6602, w6600, w6601, w6599, w6598, w6597, w6596, w6595, w6594, w6593) -> (w6592:dbl[])
                      n4545 = for {
                        tunnel: w6592 -> [w6612] mode=indexing
                        tunnel: [w6611] -> w6591 mode=indexing
                        n4546 = Format Into String(format string="%#f" ("格式字符串"), w6612) -> (resulting string=w6611:string)  [unwired: 2 in, 1 out]
                      }
                      n4547 = Build Array(string[] ["总电压过高二级", "总电压过低二级", "温度过高二级", "温度过低二级", "单组电压不均衡二级", "整组电压不均衡二级", "单组温度不均衡二级", "整组温度不均衡二级", "单体电压过高二级", "单体电压过低二级", "充电电流过高二级", "放电电流过高二级", "SOC过高二级", "SOC过低二级", "内阻过大二级", "极柱温度过高二级", "SOH过低二级"], w6591) -> (w6589:string[][])
                      n4548 = Transpose 2D Array(2D array=w6589) -> (transposed array=w6587:string[][])
                    }
                    frame #3 {
                      n4549 = control-ref of="一级故障 3"() -> (w6615:refnum<vi>)
                      n4550 = property class="Clust (严格)"(reference=w6615) -> ("Value"=w6637:T10)  [unwired: 1 in, 2 out]
                      n4551 = Unbundle(w6637) -> ("总电压过高"=w6636:dbl, "整组电压不均衡"=w6631:dbl, "SOC过高"=w6624:dbl, "单体电压过高"=w6627:dbl, "总电压过低"=w6635:dbl, "温度过高"=w6634:dbl, "温度过低"=w6633:dbl, "单组电压不均衡"=w6632:dbl, "整组温度不均衡"=w6629:dbl, "单组温度不均衡"=w6630:dbl, "单体电压过低"=w6628:dbl, "充电电流过高"=w6626:dbl, "放电电流过高"=w6625:dbl, "SOC过低"=w6623:dbl, "内阻过大"=w6622:dbl, "极柱温度过高"=w6621:dbl, "SOH过低"=w6620:dbl)
                      n4552 = Build Array(w6636, w6635, w6634, w6633, w6632, w6631, w6630, w6629, w6627, w6628, w6626, w6625, w6624, w6623, w6622, w6621, w6620) -> (w6619:dbl[])
                      n4553 = for {
                        tunnel: w6619 -> [w6639] mode=indexing
                        tunnel: [w6638] -> w6618 mode=indexing
                        n4554 = Format Into String(format string="%#f" ("格式字符串"), w6639) -> (resulting string=w6638:string)  [unwired: 2 in, 1 out]
                      }
                      n4555 = Build Array(string[] ["总电压过高三级", "总电压过低三级", "温度过高三级", "温度过低三级", "单组电压不均衡三级", "整组电压不均衡三级", "单组温度不均衡三级", "整组温度不均衡三级", "单体电压过高三级", "单体电压过低三级", "充电电流过高三级", "放电电流过高三级", "SOC过高三级", "SOC过低三级", "内阻过大三级", "极柱温度过高三级", "SOH过低三级"], w6618) -> (w6616:string[][])
                      n4556 = Transpose 2D Array(2D array=w6616) -> (transposed array=w6614:string[][])
                    }
                    frame #4 {
                      n4557 = control-ref of="加热控制参数"() -> (w6652:refnum<vi>)
                      n4558 = property class="Clust (严格)"(reference=w6652) -> ("Value"=w6651:T11)  [unwired: 1 in, 2 out]
                      n4559 = Unbundle(w6651) -> ("风机开启温度"=w6650:dbl, "风机关闭温度"=w6649:dbl, "加热开启温度"=w6648:dbl, "加热关闭温度"=w6647:dbl, "风机开启温差"=w6646:dbl, "风机关闭温差"=w6645:dbl, "加热关闭温差"=w6641:dbl)
                      n4560 = Build Array(w6650, w6649, w6648, w6647, w6646, w6645, w6641) -> (w6644:dbl[])
                      n4561 = for {
                        tunnel: w6644 -> [w6654] mode=indexing
                        tunnel: [w6653] -> w6642 mode=indexing
                        n4562 = Format Into String(format string="%#f" ("格式字符串"), w6654) -> (resulting string=w6653:string)  [unwired: 2 in, 1 out]
                      }
                    }
                    frame #5 {
                      n4563 = control-ref of="充电控制参数"() -> (w6672:refnum<vi>)
                      n4564 = property class="Clust (严格)"(reference=w6672) -> ("Value"=w6674:T12)  [unwired: 1 in, 2 out]
                      n4565 = Unbundle(w6674) -> ("最大允许单体电压"=w6671:dbl, "最大允许总电压"=w6670:dbl, "最小允许单体电压"=w6669:dbl, "最大允许充电电流"=w6668:dbl, "最小允许充电电流"=w6667:dbl, "最大允许充电温度"=w6666:dbl, "最小允许充电温度"=w6665:dbl, "电流步长"=w6664:dbl)
                      n4566 = Build Array(w6671, w6670, w6669, w6668, w6667, w6666, w6665, w6664) -> (w6673:dbl[])
                      n4567 = for {
                        tunnel: w6673 -> [w6676] mode=indexing
                        tunnel: [w6675] -> w6658 mode=indexing
                        n4568 = Format Into String(format string="%#f" ("格式字符串"), w6676) -> (resulting string=w6675:string)  [unwired: 2 in, 1 out]
                      }
                      n4569 = Insert Into Array(array=w6659, new element=w6658) -> (w6657:string[])  [unwired: 1 in]
                      n4570 = Insert Into Array(array=w6661, new element=string[] ["最大允许单体电压", "最大允许总电压", "最小允许单体电压", "最大允许充电电流", "最小允许充电电流", "最大允许充电温度", "最小允许充电温度", "电流步长"]) -> (w6656:string[])  [unwired: 1 in]
                      n4571 = Build Array(w6656, w6657) -> (w6663:string[][])
                      n4572 = Transpose 2D Array(2D array=w6663) -> (transposed array=w6662:string[][])
                    }
                    frame #6 {
                      n4573 = control-ref of="电池信息"() -> (w6700:refnum<vi>)
                      n4574 = property class="Clust (严格)"(reference=w6700) -> ("Value"=w6703:T13)  [unwired: 1 in, 2 out]
                      n4575 = Unbundle(w6703) -> ("电池串联"=w6699:dbl, "电池并联"=w6698:dbl, "累计放电总安时"=w6696:dbl, "电池包额定容量"=w6695:dbl, "电池包额定能量(kWh)"=w6694:dbl, "电池包额定总电压"=w6693:dbl, "累计充电总安时"=w6697:dbl, "电池充满次数"=w6692:dbl, "电池放空次数"=w6691:dbl, "电池充电次数"=w6690:dbl, "电池生产日期"=w6688:string, "电池厂家"=w6687:string, "电池类型"=w6686:string, "电池包组号"=w6685:string, "电池包产权标识"=w6684:string, "电池应用车型"=w6683:string, "实际容量"=w6678:dbl)
                      n4576 = Build Array(w6688, w6687, w6686, w6685, w6684, w6683) -> (w6682:string[])
                      n4577 = Build Array(w6699, w6698, w6697, w6696, w6695, w6694, w6693, w6692, w6691, w6690, w6678) -> (w6689:dbl[])
                      n4578 = for {
                        tunnel: w6689 -> [w6705] mode=indexing
                        tunnel: [w6704] -> w6681 mode=indexing
                        n4579 = Format Into String(format string="%#f" ("格式字符串"), w6705) -> (resulting string=w6704:string)  [unwired: 2 in, 1 out]
                      }
                      n4580 = Insert Into Array(array=w6682, new element=w6681) -> (w6680:string[])  [unwired: 1 in]
                      n4581 = call <vilib>:"Unset Busy.vi"() -> ()  [unwired: 2 in, 10 out]
                      n4582 = Build Array(string[] ["电池生产日期", "电池厂商", "电池类型", "电池包组号", "电池包产权标识", "电池包应用车型", "电池串联", "电池并联", "累计充电总安时", "累计放电总安时", "电池包额定容量", "电池包额定能量", "电池包额定总电压", "电池充满次数", "电池放空次数", "电池充电次数", "实际容量"], w6680) -> (w6701:string[][])
                      n4583 = Transpose 2D Array(2D array=w6701) -> (transposed array=w6679:string[][])
                    }
                  }
                  n4584 = Insert Into Array(array=w6520, index (col)=2 ("禁用的索引 (列)"), new element #1=w6517, new element #2=w6516, new element #3=w6515, new element #4=w6514, new element #5=w6513) -> (w6518:string[][])  [unwired: 1 in]
                }
                frame "从板" {
                  n4585 = local read "从板号"() -> (w6717:u8)
                  n4586 = Number To Decimal String(number=w6717) -> (decimal integer string=w6714:string)  [unwired: 1 out]
                  n4587 = Concatenate Strings("S", w6714) -> (w6715:string)
                  n4588 = Build Array("从板号" ("元素"), w6714) -> (w6712:string[])
                  n4589 = stacked-sequence {
                    seq-local: [string[] ["风机开启温度", "风机关闭温度", "加热开启温度", "加热关闭温度", "风机开启温差", "风机关闭温差", "加热关闭温差"] _ _ _ _ _] -> [_ _ _ w6786 _ _]
                    seq-local: [w6729 _ _ _ _ _] -> [_ _ _ w6782 _ _]
                    seq-local: [_ string[] ["电压过高一级", "电压过低一级", "温度过高一级", "温度过低一级", "电压不均衡一级", "温度不均衡一级", "SOC过低一级"] _ _ _ _] -> [_ _ _ w6785 _ _]
                    seq-local: [_ w6747 _ _ _ _] -> [_ _ _ w6781 _ _]
                    seq-local: [_ _ string[] ["电压过高二级", "电压过低二级", "温度过高二级", "温度过低二级", "电压不均衡二级", "温度不均衡二级", "SOC过低二级"] _ _ _] -> [_ _ _ w6784 _ _]
                    seq-local: [_ _ w6762 _ _ _] -> [_ _ _ w6780 _ _]
                    tunnel: w6712 -> [w6742 _ _ _ _ _]
                    tunnel: [w6731 _ _ _ _ _] -> w6710
                    tunnel: [_ _ _ w6787 _ _] -> w6708
                    tunnel: [_ _ _ _ w6825 _] -> w6707
                    tunnel: [_ _ _ _ _ w6861] -> _
                    frame #0 {
                      w6722 = string[] ["", "", "", "", "", "", "", "", "", "", "  "]
                      n4590 = control-ref of="项目信息 2"() -> (w6741:refnum<vi>)
                      n4591 = property class="Tbl (严格)"(reference=w6741) -> ("Value"=w6719:string[][])  [unwired: 1 in, 2 out]
                      n4592 = control-ref of="加热控制参数"() -> (w6733:refnum<vi>)
                      n4593 = property class="Clust (严格)"(reference=w6733) -> ("Value"=w6740:T11)  [unwired: 1 in, 2 out]
                      n4594 = Unbundle(w6740) -> ("风机开启温度"=w6739:dbl, "风机关闭温度"=w6738:dbl, "加热开启温度"=w6737:dbl, "加热关闭温度"=w6736:dbl, "风机开启温差"=w6735:dbl, "风机关闭温差"=w6734:dbl, "加热关闭温差"=w6728:dbl)
                      n4595 = Build Array(w6739, w6738, w6737, w6736, w6735, w6734, w6728) -> (w6732:dbl[])
                      n4596 = for {
                        tunnel: w6732 -> [w6745] mode=indexing
                        tunnel: [w6744] -> w6729 mode=indexing
                        n4597 = Format Into String(format string="%#f" ("格式字符串"), w6745) -> (resulting string=w6744:string)  [unwired: 2 in, 1 out]
                      }
                      n4598 = Index Array(array=w6719, index (col)=0 ("禁用的索引 (列)")) -> (element=w6726:string[])  [unwired: 1 in]
                      n4599 = Index Array(array=w6719, index (col)=1 ("禁用的索引 (列)")) -> (element=w6725:string[])  [unwired: 1 in]
                      n4600 = Insert Into Array(array=w6726, new element=w6722) -> (w6724:string[])  [unwired: 1 in]
                      n4601 = Insert Into Array(array=w6725, new element=w6722) -> (w6723:string[])  [unwired: 1 in]
                      n4602 = Build Array(w6724, w6723) -> (w6720:string[][])
                      n4603 = Transpose 2D Array(2D array=w6720) -> (transposed array=w6718:string[][])
                      n4604 = Insert Into Array(array=w6718, index (row)=0 ("索引 (行)"), new element=w6742) -> (w6731:string[][])  [unwired: 1 in]
                    }
                    frame #1 {
                      n4605 = control-ref of="一级故障(从板)"() -> (w6758:refnum<vi>)
                      n4606 = property class="Clust (严格)"(reference=w6758) -> ("Value"=w6757:T15)  [unwired: 1 in, 2 out]
                      n4607 = Unbundle(w6757) -> ("电压过高"=w6756:dbl, "电压过低"=w6755:dbl, "温度过高"=w6754:dbl, "温度过低"=w6753:dbl, "电压不均衡(V)"=w6752:dbl, "温度不均衡"=w6751:dbl, "SOC过低"=w6750:dbl)
                      n4608 = Build Array(w6756, w6755, w6754, w6753, w6752, w6751, w6750) -> (w6749:dbl[])
                      n4609 = for {
                        tunnel: w6749 -> [w6760] mode=indexing
                        tunnel: [w6759] -> w6747 mode=indexing
                        n4610 = Format Into String(format string="%#f" ("格式字符串"), w6760) -> (resulting string=w6759:string)  [unwired: 2 in, 1 out]
                      }
                    }
                    frame #2 {
                      n4611 = control-ref of="二级故障(从板)"() -> (w6764:refnum<vi>)
                      n4612 = property class="Clust (严格)"(reference=w6764) -> ("Value"=w6773:T15)  [unwired: 1 in, 2 out]
                      n4613 = Unbundle(w6773) -> ("电压过高"=w6772:dbl, "电压过低"=w6771:dbl, "温度过高"=w6770:dbl, "温度过低"=w6769:dbl, "电压不均衡(V)"=w6768:dbl, "温度不均衡"=w6767:dbl, "SOC过低"=w6766:dbl)
                      n4614 = Build Array(w6772, w6771, w6770, w6769, w6768, w6767, w6766) -> (w6765:dbl[])
                      n4615 = for {
                        tunnel: w6765 -> [w6775] mode=indexing
                        tunnel: [w6774] -> w6762 mode=indexing
                        n4616 = Format Into String(format string="%#f" ("格式字符串"), w6775) -> (resulting string=w6774:string)  [unwired: 2 in, 1 out]
                      }
                    }
                    frame #3 {
                      n4617 = control-ref of="三级故障(从板)"() -> (w6788:refnum<vi>)
                      n4618 = property class="Clust (严格)"(reference=w6788) -> ("Value"=w6798:T15)  [unwired: 1 in, 2 out]
                      n4619 = Unbundle(w6798) -> ("电压过高"=w6797:dbl, "电压过低"=w6796:dbl, "温度过高"=w6795:dbl, "温度过低"=w6794:dbl, "电压不均衡(V)"=w6793:dbl, "温度不均衡"=w6792:dbl, "SOC过低"=w6791:dbl)
                      n4620 = Build Array(w6797, w6796, w6795, w6794, w6793, w6792, w6791) -> (w6790:dbl[])
                      n4621 = for {
                        tunnel: w6790 -> [w6800] mode=indexing
                        tunnel: [w6799] -> w6779 mode=indexing
                        n4622 = Format Into String(format string="%#f" ("格式字符串"), w6800) -> (resulting string=w6799:string)  [unwired: 2 in, 1 out]
                      }
                      n4623 = Insert Into Array(array=w6786, new element #1=w6785, new element #2=w6784, new element #3=string[] ["电压过高三级", "电压过低三级", "温度过高三级", "温度过低三级", "电压不均衡三级", "温度不均衡三级", "SOC过低三级"]) -> (w6777:string[])  [unwired: 1 in]
                      n4624 = Insert Into Array(array=w6782, new element #1=w6781, new element #2=w6780, new element #3=w6779) -> (w6778:string[])  [unwired: 1 in]
                      n4625 = Build Array(w6777, w6778) -> (w6789:string[][])
                      n4626 = Transpose 2D Array(2D array=w6789) -> (transposed array=w6787:string[][])
                    }
                    frame #4 {
                      n4627 = control-ref of="快换(从板)"() -> (w6824:refnum<vi>)
                      n4628 = property class="Clust (严格)"(reference=w6824) -> ("Value"=w6837:T16)  [unwired: 1 in, 2 out]
                      n4629 = Unbundle(w6837) -> ("串联数"=w6836:dbl, "并联数"=w6835:dbl, "电池厂家"=w6834:dbl, "电池类型"=w6833:dbl, "额定能量"=w6832:dbl, "额定容量"=w6831:dbl, "实际容量"=w6830:dbl, "额定总压"=w6823:dbl, "产权标识"=w6822:dbl, "应用车型"=w6821:dbl, "电池包组号"=w6820:dbl, "SOC"=w6818:dbl, "充电总安时"=w6817:dbl, "放电总安时"=w6816:dbl, "放空次数"=w6815:dbl, "充满次数"=w6814:dbl, "充电次数"=w6813:dbl, "车牌号"=w6803:string, "生产日期"=w6802:string, "最大允许单体电压"=w6812:dbl, "最大允许总电压"=w6811:dbl, "最大允许温度"=w6810:dbl, "最小允许温度"=w6809:dbl, "最大允许充电电流"=w6808:dbl, "最小允许充电电流"=w6807:dbl, "最小允许单体电压"=w6806:dbl, "电流步长"=w6805:dbl, "电池包序号"=w6804:dbl)
                      n4630 = Build Array(w6836, w6835, w6834, w6833, w6832, w6831, w6830, w6823, w6822, w6821, w6820, w6818, w6817, w6816, w6815, w6814, w6813, w6812, w6811, w6810, w6809, w6808, w6807, w6806, w6805, w6804) -> (w6829:dbl[])
                      n4631 = for {
                        tunnel: w6829 -> [w6839] mode=indexing
                        tunnel: [w6838] -> w6827 mode=indexing
                        n4632 = Format Into String(format string="%#f" ("格式字符串"), w6839) -> (resulting string=w6838:string)  [unwired: 2 in, 1 out]
                      }
                      n4633 = Insert Into Array(array=w6827, new element #1=w6803, new element #2=w6802) -> (w6819:string[])  [unwired: 1 in]
                      n4634 = call <vilib>:"Unset Busy.vi"() -> ()  [unwired: 2 in, 10 out]
                      n4635 = Build Array(string[] ["电池串联数", "电池并联数", "电池厂家", "额定能量", "额定容量", "实际容量", "额定总压", "产权标识", "应用车型", "电池包组号", "SOC", "充电总安时", "放电总安时", "放空次数", "充满次数", "充电次数", "最大允许单体电压", "最大允许总电压", "最大允许温度", "最小允许温度", "最大允许充电电流", "最小允许充电电流", "最小允许单体电压", "电流步长", "电池包序号"], w6819) -> (w6828:string[][])
                      n4636 = Transpose 2D Array(2D array=w6828) -> (transposed array=w6825:string[][])
                    }
                    frame #5 {
                      n4637 = local read "均衡参数"() -> (w6860:T17)
                      n4638 = Unbundle(w6860) -> ("充电结束电压(90%)"=w6852:sgl, "充电结束电压(91%)"=w6851:sgl, "充电结束电压(92%)"=w6850:sgl, "充电结束电压(93%)"=w6849:sgl, "充电结束电压(94%)"=w6848:sgl, "均衡计算-电压高阀值1级"=w6859:sgl, "均衡计算-电压高阀值2级"=w6858:sgl, "均衡计算-电压低阀值1级"=w6857:sgl, "均衡计算-电压低阀值2级"=w6856:sgl, "均衡计算-最低电压阀值"=w6855:sgl, "均衡停止-最低电压阀值"=w6854:sgl, "均衡计算-电压极差阀值"=w6853:sgl, "充电结束电压(95%)"=w6847:sgl, "充电结束电压(96%)"=w6846:sgl, "充电结束电压(97%)"=w6845:sgl, "充电结束电压(98%)"=w6844:sgl, "充电结束电压(99%)"=w6843:sgl, "充电结束电压(100%)"=w6842:sgl)
                      n4639 = Build Array(w6859, w6858, w6857, w6856, w6855, w6854, w6853, w6852, w6851, w6850, w6849, w6848, w6847, w6846, w6845, w6844, w6843, w6842) -> (w6864:sgl[])
                      n4640 = for {
                        tunnel: w6864 -> [w6866] mode=indexing
                        tunnel: [w6865] -> w6841 mode=indexing
                        n4641 = Format Into String(format string="%#f" ("格式字符串"), w6866) -> (resulting string=w6865:string)  [unwired: 2 in, 1 out]
                      }
                      n4642 = call <vilib>:"Unset Busy.vi"() -> ()  [unwired: 2 in, 10 out]
                      n4643 = Build Array(string[] ["均衡计算-电压高阀值1级", "均衡计算-电压高阀值2级", "均衡计算-电压低阀值1级", "均衡计算-电压低阀值2级", "均衡计算-最低电压阀值", "均衡停止-最低电压阀值", "均衡计算-电压极差阀值", "充电结束电压(90%)", "充电结束电压(91%)", "充电结束电压(92%)", "充电结束电压(93%)", "充电结束电压(94%)", "充电结束电压(95%)", "充电结束电压(96%)", "充电结束电压(97%)", "充电结束电压(98%)", "充电结束电压(99%)", "充电结束电压(100%)"], w6841) -> (w6863:string[][])
